vi "Write Accounts Data.vi"(8 "error in":errorcluster, 11 "Accounts":T1[](array[typedef])) -> (0 "error out":errorcluster)   [LabVIEW 2019, in "Configuration Database.lvlib"]
doc: "Overrides accounts data from data in memory."
uses:
  Configuration Database.lvlib
  Typedefs/Account.ctl
panel:
  # "[Covers: CD1A]"
  # "[Covers: CD1B]"
  # "[Covers: CD1C]"
  # "[Covers: CD1D]"
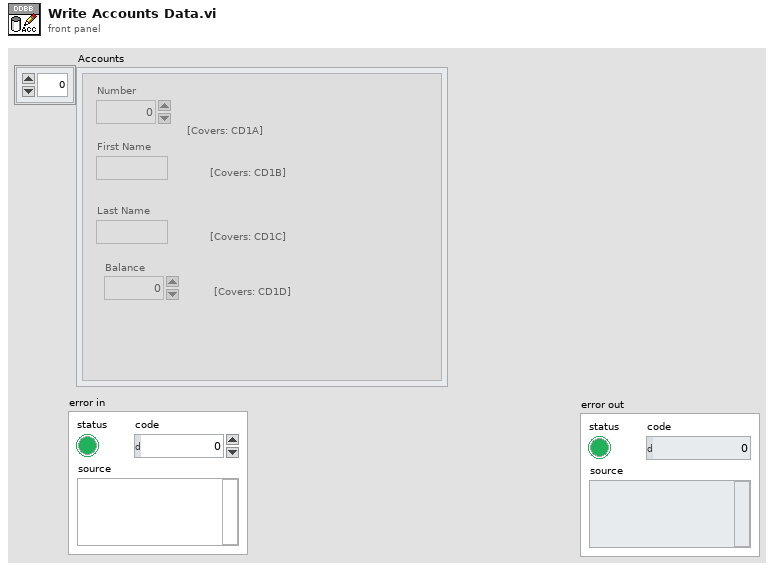
[diagram p1: front panel]
types:
  T1 = typedef "Configuration Database.lvlib/Account.ctl" = cluster{"Number":i32, "First Name":string, "Last Name":string, "Balance":dbl}
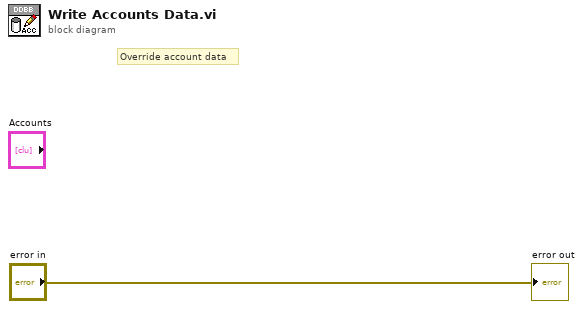
[diagram p0: block diagram]
diagram:
  # "Override account data"
  "error out" <- "error in"
